vi "1D bead separation calculation.vi"(0 "Trap 1 Bead Size (nm)":dbl=810.0, 1 "Trap 2 Bead Size (nm)":dbl=810.0, 2 "Trap 3 Bead Size (nm)":dbl=810.0, 3 "Absolute Positions":waveform(dbl)[](array[waveform]), 4 "Pair choice":enum16{"1-2", "2-3", "3-1"}(ring)) -> (5 "Output separation":dbl[](array[numeric]), 6 "Output waveforms":waveform(dbl)[](array[waveform]))   [LabVIEW 2014]
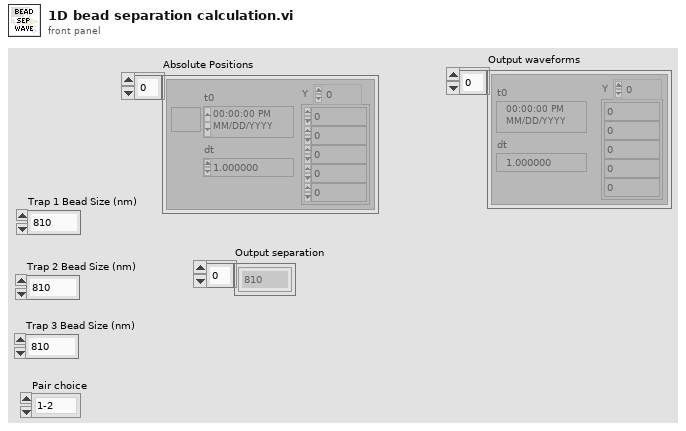
[diagram p1: front panel]
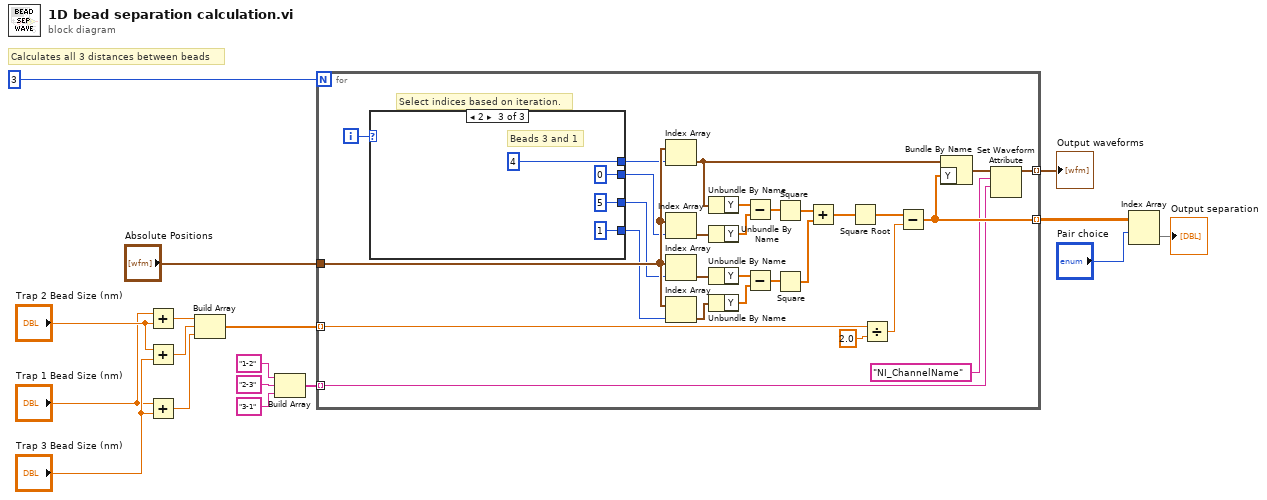
[diagram p0: block diagram]
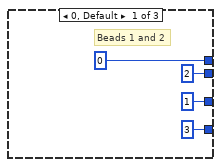
[diagram p2: hidden frame]
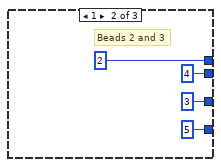
[diagram p3: hidden frame]
diagram:
  # "Calculates all 3 distances between beads"
  n1 = Add(x="Trap 1 Bead Size (nm)", y="Trap 2 Bead Size (nm)") -> (x+y=w8:dbl)
  n2 = Add(x="Trap 2 Bead Size (nm)", y="Trap 3 Bead Size (nm)") -> (x+y=w7:dbl)
  n3 = Add(x="Trap 1 Bead Size (nm)", y="Trap 3 Bead Size (nm)") -> (x+y=w6:dbl)
  n4 = Build Array(w8, w7, w6) -> (w5:dbl[])
  n5 = Build Array("1-2", "2-3", "3-1") -> (w1:string[])
  n6 = for {
    N: 3 -> [_]
    tunnel: "Absolute Positions" -> [w44]
    tunnel: [w20] -> w16 mode=indexing
    tunnel: [w24] -> w14 mode=indexing
    tunnel: w5 -> [w23] mode=indexing
    tunnel: w1 -> [w19] mode=indexing
    i -> [w45]
    # "Select indices based on iteration."
    n7 = case shown="2" w45 {
      tunnel: [0 2 4] -> w43
      tunnel: [2 4 0] -> w42
      tunnel: [1 3 5] -> w41
      tunnel: [3 5 1] -> w40
      frame 0, Default {
        # "Beads 1 and 2"
      }
      frame 1 {
        # "Beads 2 and 3"
      }
      frame 2 {
        # "Beads 3 and 1"
      }
    }
    n8 = Index Array(array=w44, index=w43) -> (element=w27:waveform(dbl))
    n9 = Index Array(array=w44, index=w42) -> (element=w39:waveform(dbl))
    n10 = Index Array(array=w44, index=w41) -> (element=w38:waveform(dbl))
    n11 = Index Array(array=w44, index=w40) -> (element=w37:waveform(dbl))
    n12 = Unbundle By Name(w27) -> ("Y"=w35:dbl[])
    n13 = Unbundle By Name(w39) -> ("Y"=w36:dbl[])
    n14 = Unbundle By Name(w38) -> ("Y"=w34:dbl[])
    n15 = Unbundle By Name(w37) -> ("Y"=w33:dbl[])
    n16 = Subtract(x=w35, y=w36) -> (x-y=w32:dbl[])
    n17 = Subtract(x=w34, y=w33) -> (x-y=w31:dbl[])
    n18 = Square(x=w32) -> (x^2=w30:dbl[])
    n19 = Square(x=w31) -> (x^2=w29:dbl[])
    n20 = Add(x=w30, y=w29) -> (x+y=w28:dbl[])
    n21 = Square Root(x=w28) -> (sqrt(x)=w25:dbl[])
    n22 = Divide(x=w23, y=2.0) -> (x/y=w22:dbl)
    n23 = Subtract(x=w25, y=w22) -> (x-y=w24:dbl[])
    n24 = Bundle By Name(cluster=w27, "Y"=w24) -> (w21:waveform(dbl))
    n25 = Set Waveform Attribute(5:w19, 6:"NI_ChannelName", 7:w21) -> (3:w20:waveform(dbl))  [unwired: 1 in, 2 out]
  }
  "Output waveforms" <- w16
  n26 = Index Array(array=w14, index (row)="Pair choice") -> (element=→"Output separation":dbl[])  [unwired: 1 in]
